vi "acquisitionAcquireVolumeFindNeurons.vi"(3 "piezoPosition":dbl[](array[numeric]), 4 "hamamatsuFrameCounter":u32[](array[numeric]), 5 "frameAvailable":i32[](array[numeric]), 6 "volumeFirstFrame":u32[](array[numeric])) -> (0 "XY":u16[][][](array[numeric]), 1 "XYZ":dbl[][](array[numeric]), 2 "volume out":u16[][][](array[numeric]))   [LabVIEW 2017]
uses:
  opencvSegmentConvertCoordinates-multiFrames.vi
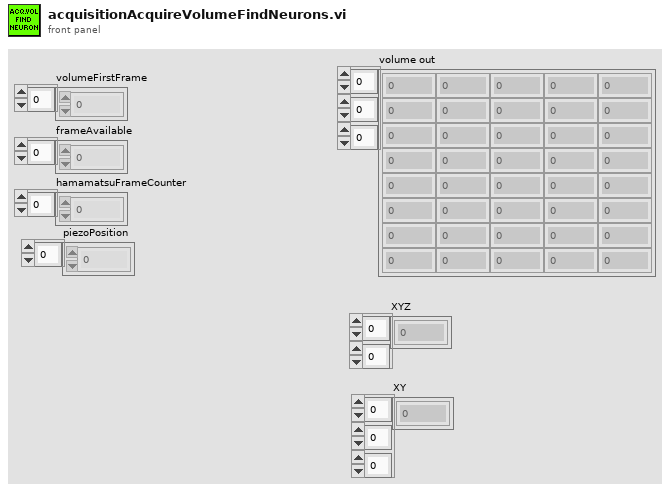
[diagram p1: front panel]
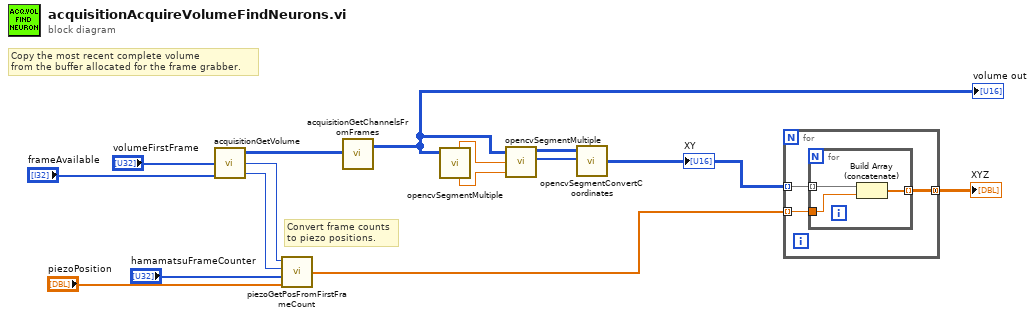
[diagram p0: block diagram]
diagram:
  # "Convert frame counts\nto piezo positions."
  # "Copy the most recent complete volume\nfrom the buffer allocated for the frame grabber."
  n1 = call "acquisitionGetVolume.vi"("frameAvailable"="frameAvailable", "volumeFirstFrame"="volumeFirstFrame") -> ("numberOfFrames"=w14:u32, "absoluteCountFirstFrame"=w15:u32, "volume out"=w7:u16[][][])  [unwired: 1 in]
  n2 = call "piezoGetPosFromFirstFrameCount.vi"("piezoPosition"="piezoPosition", "hamamatsuFrameCounter"="hamamatsuFrameCounter", "numberOfFrames"=w14, "firstFrameCount"=w15) -> ("piezo pos out"=w13:dbl[])  [unwired: 2 in]
  n3 = call "acquisitionGetChannelsFromFrames.vi"("frameIn"=w7) -> ("Red"=w6:u16[][][])  [unwired: 1 out]
  "volume out" <- w6
  n4 = call "opencvSegmentMultiple.vi"("ImgIn"=w6) -> ("maxY"=w3:dbl, "maxX"=w2:dbl)  [unwired: 2 in, 4 out]
  n5 = call "opencvSegmentMultiple.vi"("maxYInStack"=w3, "maxXInStack"=w2, "ImgIn"=w6) -> ("NeuronN[frame]"=w5:u16[], "NeuronXY[frame]"=w4:u16[][])  [unwired: 4 out]
  n6 = call-poly "opencvSegmentConvertCoordinates.vi"("NeuronN"=w5, "NeuronXY"=w4) -> ("XY"=w1:u16[][][])  [unwired: 1 in]
  "XY" <- w1
  n7 = for {
    tunnel: w1 -> [w18] mode=indexing
    tunnel: w13 -> [w17] mode=indexing
    tunnel: [w16] -> w12 mode=concatenating
    n8 = for {
      tunnel: w18 -> [w21] mode=indexing
      tunnel: w17 -> [w20]
      tunnel: [w19] -> w16 mode=indexing
      n9 = Build Array (concatenate)(w21, w20) -> (w19:dbl[])
    }
  }
  "XYZ" <- w12
